vi "Teleop.vi"(10 "Match Info":T1={"Autonomous Elapsed Seconds"=0.0, "TeleOp Elapsed Seconds"=0.0, "Disabled Elapsed Seconds"=0.0, "Visited Autonomous"=FALSE, "Visited TeleOp"=FALSE, "Visited Disabled"=FALSE, "Autonomous Settings"={"Autonomous Style"=enum."Independent", "VI Refnum"=refnum}}, 11 "Call Context":T2) -> ()   [LabVIEW 2014]
doc: "This VI is called for each TeleOp packet received from the DS where the robot is not disabled. It is often used to read from the joysticks and update I/O or to update setpoints for timed control loops. It should complete and return within 20 milliseconds or it may miss DS packets."
uses:
  <vilib>/Rock Robotics/WPI/DriverStation/WPI_DriverStationDerivedRobotMode.ctl
  <vilib>/Rock Robotics/WPI/DriverStation/WPI_DriverStationMatch Info.ctl
  <vilib>/Rock Robotics/WPI/Joystick/WPI_JoystickGetSetRefNum.vi
  TORC Code/GlobalVariable.vi
  <vilib>/Rock Robotics/Network Tables/SD Read Boolean.vi
  <vilib>/Rock Robotics/Network Tables/SD Read Number.vi
panel:
  out "Sample Slider 0":dbl(slide) scale=0.0..5.0
  out "Sample Boolean 1":bool
  out "Sample Boolean 0":bool
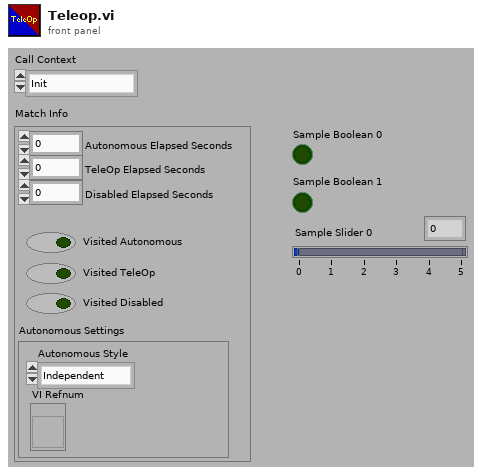
[diagram p1: front panel]
types:
  T1 = typedef "WPI_DriverStationMatch Info.ctl" = cluster{"Autonomous Elapsed Seconds":dbl, "TeleOp Elapsed Seconds":dbl, "Disabled Elapsed Seconds":dbl, "Visited Autonomous":bool, "Visited TeleOp":bool, "Visited Disabled":bool, "Autonomous Settings":cluster{"Autonomous Style":enum16{"Iterative", "Independent"}, "VI Refnum":refnum<vi>}}
  T2 = typedef "WPI_DriverStationDerivedRobotMode.ctl" = enum16{"Init", "Execute", "Stop"}
  T3 = typedef "WPI_JoystickDevRef.ctl" = cluster{"Device":T4}
  T4 = typedef "WPI_JoystickDeviceEnum.ctl" = enum16{"USB 0", "USB 1", "USB 2", "USB 3", "USB 4", "USB 5"}
  T5 = cluster{"Buttons[0]":bool, "Buttons[1]":bool, "Buttons[2]":bool, "Buttons[3]":bool, "Buttons[4]":bool, "Buttons[5]":bool, "Buttons[6]":bool, "Buttons[7]":bool, "Buttons[8]":bool}
  T6 = cluster{"Axes[0]":dbl, "Axes[1]":dbl, "Axes[2]":dbl, "Axes[3]":dbl, "Axes[4]":dbl, "Axes[5]":dbl, "Axes[6]":dbl, "Axes[7]":dbl, "Axes[8]":dbl}
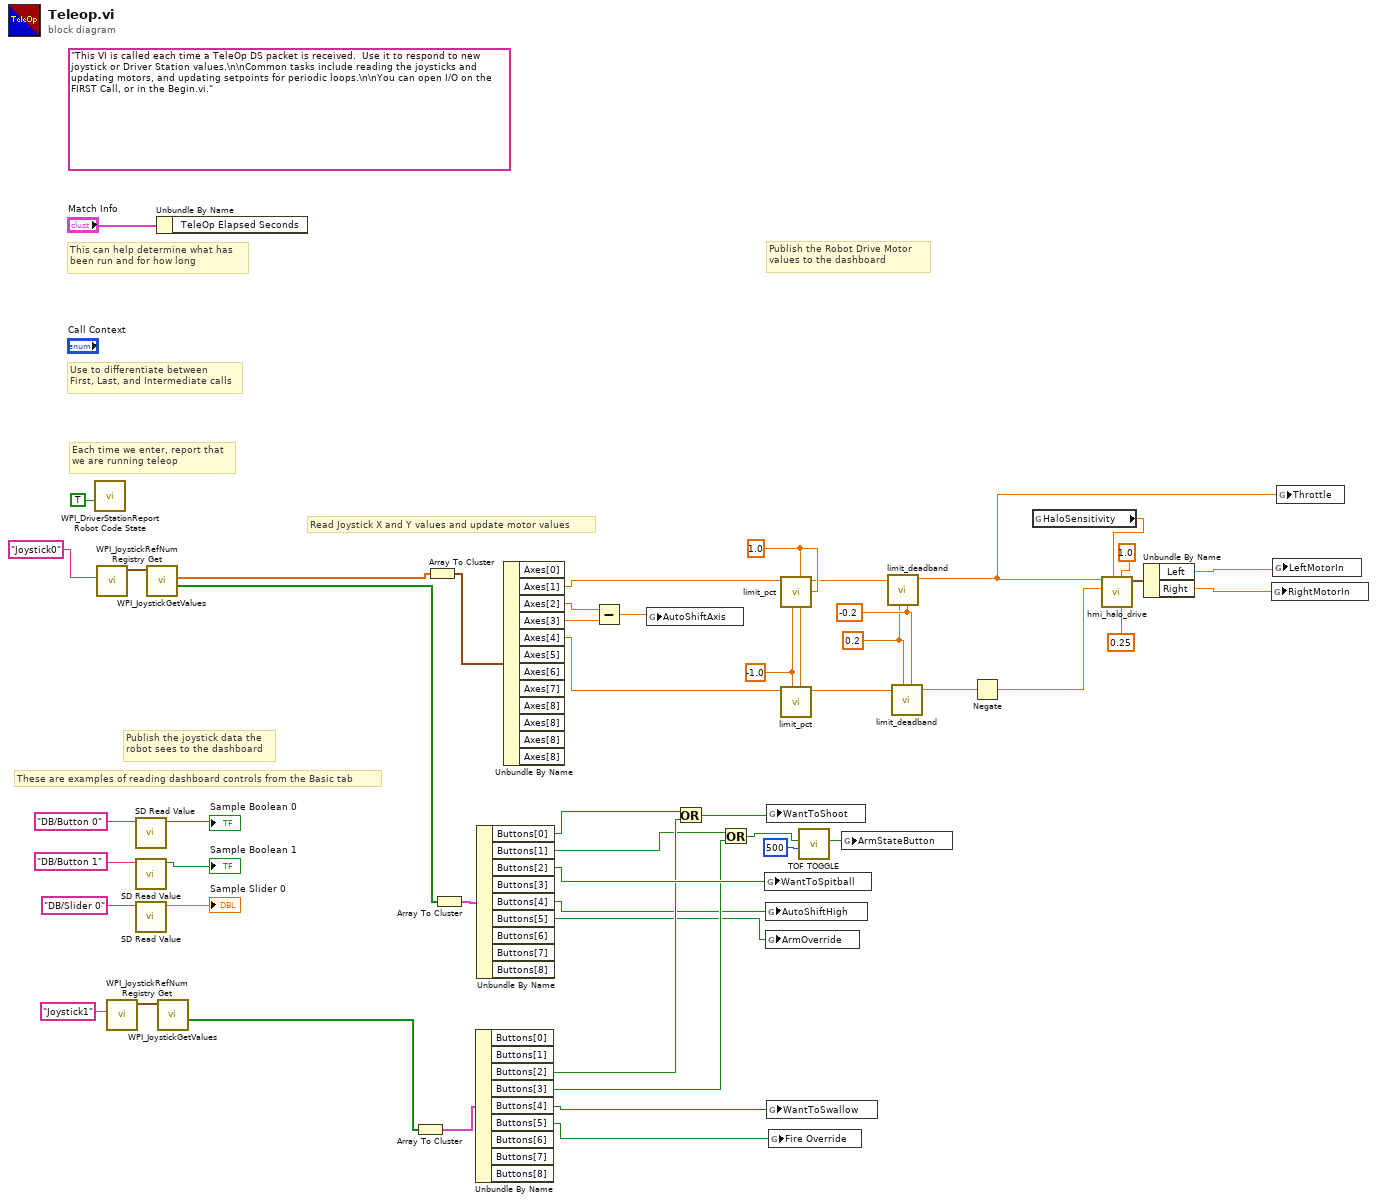
[diagram p0: block diagram]
diagram:
  w36 = 1.0 ("upper limit")
  w35 = -1.0 ("lower limit")
  w29 = -0.2 ("lower limit")
  w28 = 0.2 ("upper limit")
  (unwired) "This VI is called each time a TeleOp DS packet is received.  Use it to respond to new joystick or Driver Station values.\n\nCommon tasks include reading the joysticks and updating motors, and updating setpoints for periodic loops.\n\nYou can open I/O on the FIRST Call, or in the Begin.vi."
  # "These are examples of reading dashboard controls from the Basic tab"
  # "Publish the Robot Drive Motor\nvalues to the dashboard"
  # "Publish the joystick data the\nrobot sees to the dashboard"
  # "Each time we enter, report that\nwe are running teleop"
  # "Use to differentiate between\nFirst, Last, and Intermediate calls"
  # "This can help determine what has\nbeen run and for how long"
  # "Read Joystick X and Y values and update motor values"
  n1 = call <vilib>:"WPI_DriverStationReport Robot Code State.vi"("TeleOp"=TRUE ("Autonomous")) -> ()  [unwired: 10 in, 1 out]
  n2 = call <vilib>:"WPI_JoystickRefNum Registry Get.vi"("refnum name"="Joystick0") -> ("JoystickDevRef"=w49:T3)  [unwired: 1 in, 9 out]
  n3 = call <vilib>:"WPI_JoystickRefNum Registry Get.vi"("refnum name"="Joystick1") -> ("JoystickDevRef"=w17:T3)  [unwired: 1 in, 9 out]
  n4 = call-poly <vilib>:"SD Read Value.vi"("Name"="DB/Button 0" ("refnum name")) -> ("Boolean"=→"Sample Boolean 0":bool)  [unwired: 8 in, 2 out]
  n5 = call-poly <vilib>:"SD Read Value.vi"("Name"="DB/Button 1" ("refnum name")) -> ("Boolean"=→"Sample Boolean 1":bool)  [unwired: 8 in, 2 out]
  n6 = call-poly <vilib>:"SD Read Value.vi"("Name"="DB/Slider 0" ("refnum name")) -> ("Numeric"=→"Sample Slider 0":dbl)  [unwired: 8 in, 2 out]
  n7 = call <vilib>:"WPI_JoystickGetValues.vi"("JoystickDevRef"=w49) -> ("Buttons"=w39:bool[], "Axes"=w41:dbl[])  [unwired: 6 in, 3 out]
  n8 = Unbundle By Name("Match Info") -> ()  [unwired: 1 out]
  n9 = call <vilib>:"WPI_JoystickGetValues.vi"("JoystickDevRef"=w17) -> ("Buttons"=w1:bool[])  [unwired: 6 in, 4 out]
  n10 = Array To Cluster(array=w1) -> (cluster=w16:T5)
  n11 = Array To Cluster(array=w41) -> (cluster=w40:T6)
  n12 = Array To Cluster(array=w39) -> (cluster=w38:T5)
  n13 = Unbundle By Name(w16) -> ("Buttons[0]"=w14:bool, "Buttons[1]"=w11:bool, "Buttons[2]"=w9:bool, "Buttons[3]"=w8:bool)  [unwired: 5 out]
  n14 = Unbundle By Name(w38) -> ("Buttons[0]"=w15:bool, "Buttons[1]"=w10:bool, "Buttons[2]"=w19:bool, "Buttons[4]"=w7:bool, "Buttons[5]"=w6:bool)  [unwired: 4 out]
  n15 = Unbundle By Name(w40) -> ("Axes[1]"=w23:dbl, "Axes[2]"=w4:dbl, "Axes[3]"=w3:dbl, "Axes[4]"=w22:dbl)  [unwired: 8 out]
  n16 = Subtract(x=w4, y=w3) -> (x-y=w2:dbl)
  n17 = global write "GlobalVariable.vi" "AutoShiftAxis"(w2) -> ()
  n18 = Or(x=w15, y=w14) -> (x .or. y?=w13:bool)
  n19 = Or(x=w10, y=w11) -> (x .or. y?=w12:bool)
  n20 = global write "GlobalVariable.vi" "WantToSpitball"(w19) -> ()
  n21 = global write "GlobalVariable.vi" "AutoShiftHigh"(w7) -> ()
  n22 = global write "GlobalVariable.vi" "ArmOverride"(w6) -> ()
  n23 = global write "GlobalVariable.vi" "WantToShoot"(w13) -> ()
  n24 = global write "GlobalVariable.vi" "WantToSwallow"(w9) -> ()
  n25 = global write "GlobalVariable.vi" "Fire Override"(w8) -> ()
  n26 = call "limit_pct.vi"("upper limit"=w36, "lower limit"=w35, "PCT"=w23) -> ("PCT Out"=w33:dbl)  [unwired: 8 in]
  n27 = call "limit_pct.vi"("upper limit"=w36, "lower limit"=w35, "PCT"=w22) -> ("PCT Out"=w34:dbl)  [unwired: 8 in]
  n28 = call "TOF TOGGLE.vi"("Delay (ms)"=u32 500 ("Delay ms"), "Input"=w12) -> ("Output"=w21:bool)  [unwired: 9 in]
  n29 = global write "GlobalVariable.vi" "ArmStateButton"(w21) -> ()
  n30 = call "limit_deadband.vi"("lower limit"=w29, "upper limit"=w28, "Val"=w33) -> ("Val Out"=w24:dbl)  [unwired: 8 in]
  n31 = call "limit_deadband.vi"("lower limit"=w29, "upper limit"=w28, "Val"=w34) -> ("Val Out"=w27:dbl)  [unwired: 8 in]
  n32 = Negate(x=w27) -> (-x=w32:dbl)
  n33 = global read "GlobalVariable.vi" "HaloSensitivity"() -> (w37:dbl)
  n34 = call "hmi_halo_drive.vi"("QuickTurn Const"=0.25, "Quickturn_Sens_Low"=1.0 ("QuickTurn Const"), "Speedturn_Sens_Low"=w37, "Wheel"=w32, "Throttle"=w24) -> ("Drive Data"=w5:cluster{"Left":dbl, "Right":dbl})  [unwired: 6 in]
  n35 = Unbundle By Name(w5) -> ("Left"=w25:dbl, "Right"=w26:dbl)
  n36 = global write "GlobalVariable.vi" "RightMotorIn"(w26) -> ()
  n37 = global write "GlobalVariable.vi" "LeftMotorIn"(w25) -> ()
  n38 = global write "GlobalVariable.vi" "Throttle"(w24) -> ()
